vi "TestMBcode.vi"() -> ()   [LabVIEW 2020]
uses:
  <vilib>/Modbus/master/Create Master Instance (Serial).vi
  <vilib>/Modbus/master/Modbus Master.lvclass
panel:
  out "register values":u16[](array[numeric])
  in  "starting address":u16
  in  "number of holding registers":u16
  in  "baud rate (9600)":u32=9600
  in  "serial type":enum16{"RTU", "ASCII"}(ring)
  in  "unit ID":u8=1
  in  "VISA resource name":refnum<visa-resource-name>
  out "error out":errorcluster
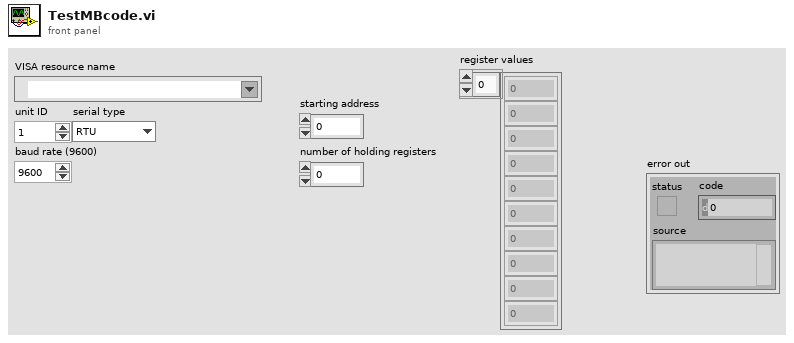
[diagram p1: front panel]
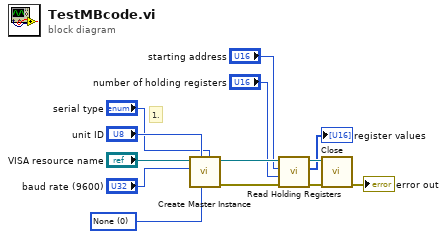
[diagram p0: block diagram]
diagram:
  w4 = u16 0 items=["None", "Odd", "Even"] ("parity (Even)")
  # "1."
  n1 = call-poly <vilib>:"Create Master Instance.vi"("serial type"="serial type", "parity (Even)"=w4, "unit ID"="unit ID", "baud rate (9600)"="baud rate (9600)", "VISA resource name"="VISA resource name") -> ("error out"=w12:errorcluster, "serial master instance"=w13:refnum<class "Modbus Master.lvclass">)  [unwired: 5 in]
  n2 = call-dynamic "Read Holding Registers.vi"("error in (no error)"=w12, "number of holding registers"="number of holding registers", "starting address"="starting address", "Modbus master in"=w13) -> ("error out"=w10:errorcluster, "register values"=→"register values":u16[], "Modbus master out"=w11:refnum<class "Modbus Master.lvclass">)  [unwired: 5 in]
  n3 = call-dynamic "Close.vi"("error in (no error)"=w10, "Modbus master in"=w11) -> ("error out"=→"error out":errorcluster)  [unwired: 9 in]
